vi "Read Base Path.vi"(8 "error in (no error)":errorcluster, 11 "Generic Test Stand in":refnum<class "Generic Test Stand.lvclass">) -> (0 "error out":errorcluster, 2 "Base Path":path, 3 "Generic Test Stand out":refnum<class "Generic Test Stand.lvclass">)   [LabVIEW 2019, in "Generic Test Stand.lvclass"]
uses:
  Generic Test Stand.lvclass
  Generic Test Stand.lvclass/Generic Test Stand.ctl
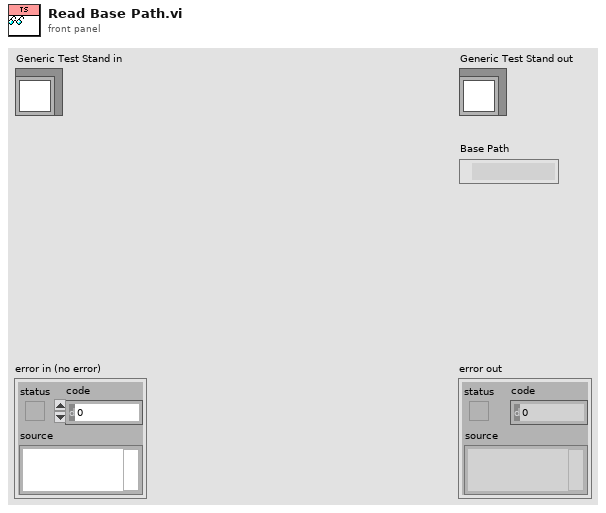
[diagram p1: front panel]
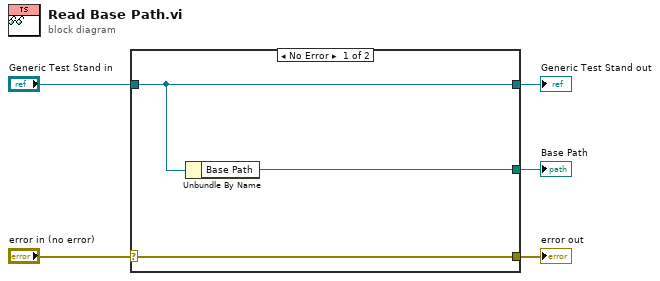
[diagram p0: block diagram]
diagram:
  n1 = case shown="No Error" "error in (no error)" {
    selector: "error in (no error)" -> [w8 w9]
    tunnel: [w8 w9] -> w4
    tunnel: [w7 w10] -> w2
    tunnel: "Generic Test Stand in" -> [w7 w10]
    tunnel: [w6 _] -> w1
    frame No Error {
      n2 = Unbundle By Name(w7) -> ("Base Path"=w6:path)
    }
    frame Error {
    }
  }
  "error out" <- w4
  "Generic Test Stand out" <- w2
  "Base Path" <- w1
